vi "MICROMATIC.vi"() -> ()   [LabVIEW 2019]
uses:
  <vilib>/Utility/file.llb/Write Delimited Spreadsheet (string).vi
panel:
  in  "DATA LOGGING":bool
  in  "TEMPERATURE":bool
  out "DATE & TIME":timestamp
  out "Temperature (°C )":dynamicdata(graph)
  in  "SELECT A .CSV FILE TO WRITE DATA":path
  out "Vibration ( µA)":dynamicdata(graph)
  in  "VIBRATION":bool
  # "1.Connect vibration sensor to NI-9234 placed in slot no 2 of NI C-DAQ\n2.Connect RTD sensor to NI-9211 placed in slot no 3 of NI C-DAQ"
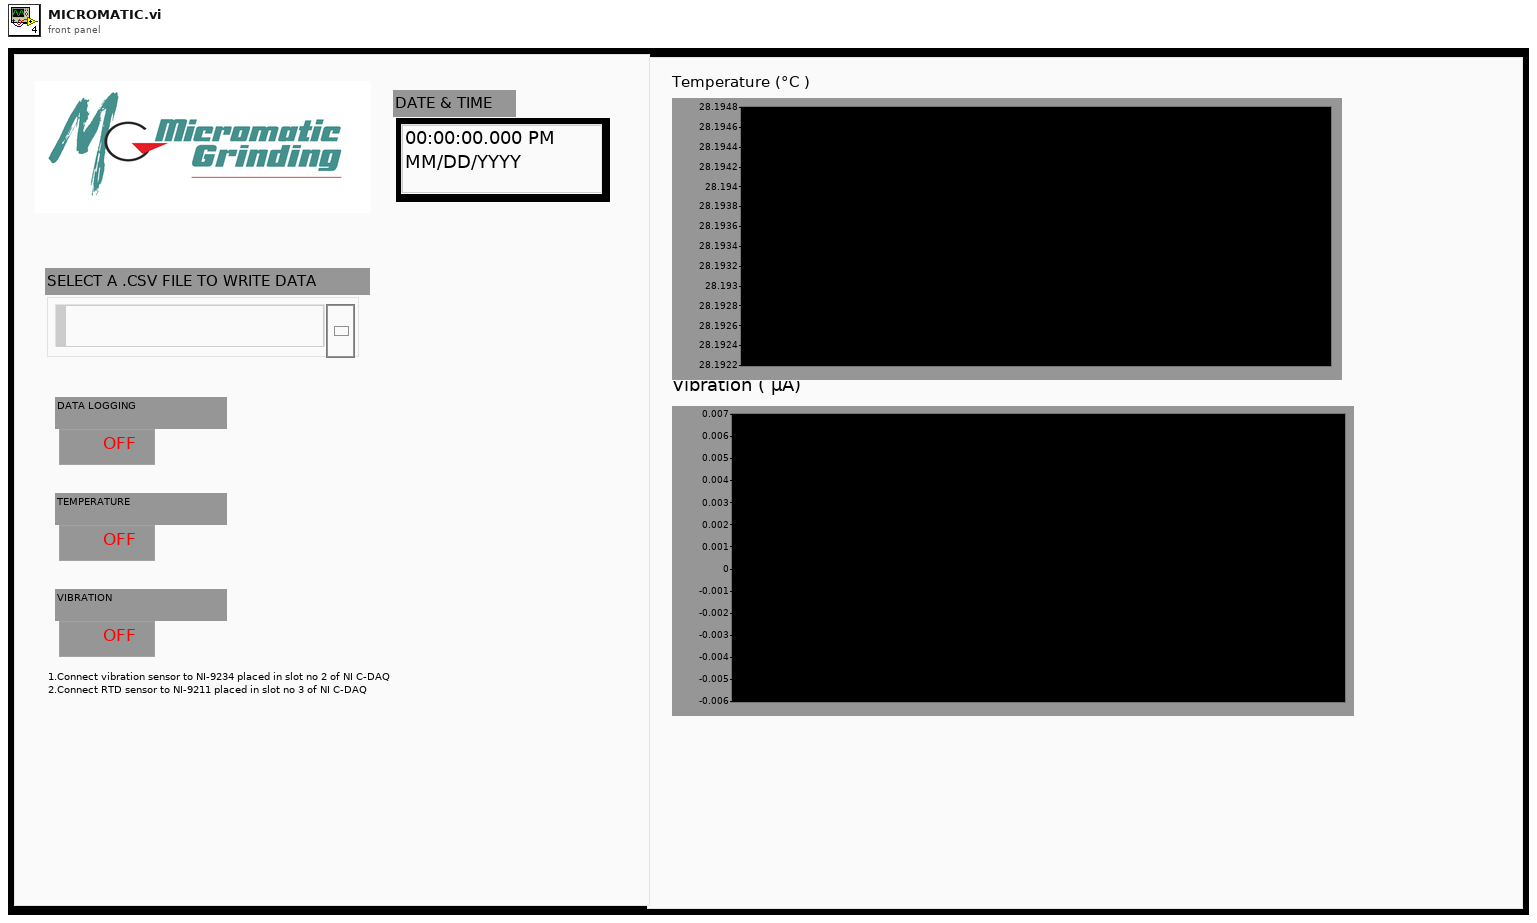
[diagram p1: front panel]
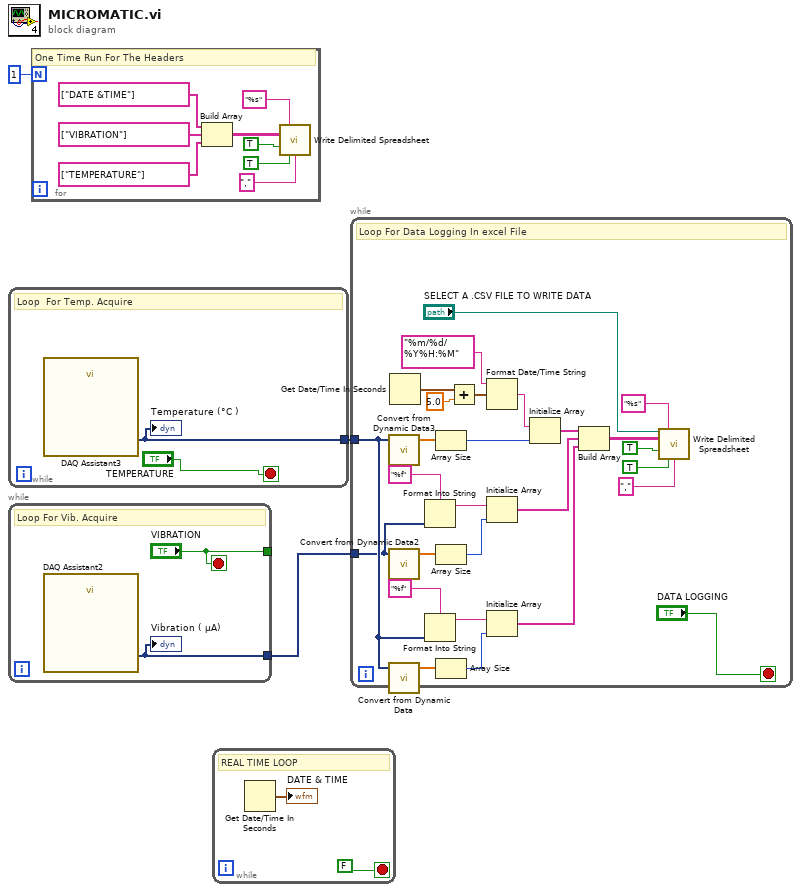
[diagram p0: block diagram]
diagram:
  n1 = while {
    tunnel: [w5] -> w1
    stop <- "TEMPERATURE" stop-if-true
    # "Loop  For Temp. Acquire"
    n2 = call "DAQ Assistant3"() -> ("data"=w5:dynamicdata)  [unwired: 16 in, 3 out]
    "Temperature (°C )" <- w5
  }
  n3 = while {
    tunnel: [w7] -> w2
    tunnel: ["VIBRATION"] -> _
    stop <- "VIBRATION" stop-if-true
    # "Loop For Vib. Acquire"
    n4 = call "DAQ Assistant2"() -> ("data"=w7:dynamicdata)  [unwired: 16 in, 3 out]
    "Vibration ( µA)" <- w7
  }
  n5 = for {
    N: 1 -> [_]
    # "One Time Run For The Headers"
    n6 = Build Array(string[] ["DATE &TIME"], string[] ["VIBRATION"], string[] ["TEMPERATURE"]) -> (w11:string[][])
    n7 = call-poly <vilib>:"Write Delimited Spreadsheet.vi"("format (%s)"="%s", "2D data"=w11, "append to file? (new file:F)"=TRUE, "transpose? (no:F)"=TRUE, "delimiter (\\t)"="," ("delimiter (\\t)")) -> ()  [unwired: 9 in, 2 out]
  }
  n8 = while {
    stop <- FALSE ("TIME") stop-if-true
    # "REAL TIME LOOP"
    n9 = Get Date/Time In Seconds() -> (seconds since 1Jan1904=→"DATE & TIME":timestamp)
  }
  n10 = while {
    tunnel: w1 -> [w20]
    tunnel: w2 -> [w19]
    stop <- "DATA LOGGING" stop-if-true
    # "Loop For Data Logging In excel File"
    n11 = call "Convert from Dynamic Data3"("Dynamic Data Type"=w20) -> ("Array"=w28:dbl[])  [unwired: 3 in]
    n12 = call "Convert from Dynamic Data2"("Dynamic Data Type"=w19) -> ("Array"=w39:dbl[])  [unwired: 3 in]
    n13 = call "Convert from Dynamic Data"("Dynamic Data Type"=w20) -> ("Array"=w41:dbl[])  [unwired: 3 in]
    n14 = Get Date/Time In Seconds() -> (seconds since 1Jan1904=w23:timestamp)
    n15 = Format Into String(format string="%f", w19) -> (resulting string=w38:string)  [unwired: 2 in, 1 out]
    n16 = Format Into String(format string="%f", w20) -> (resulting string=w42:string)  [unwired: 2 in, 1 out]
    n17 = Array Size(array=w28) -> (size(s)=w27:i32)
    n18 = Array Size(array=w39) -> (size(s)=w37:i32)
    n19 = Array Size(array=w41) -> (size(s)=w40:i32)
    n20 = Add(x=w23, y=5.0) -> (x+y=w21:timestamp)
    n21 = Format Date/Time String(time format string (%c)="%m/%d/%Y%H:%M", seconds (now)=w21) -> (date/time string=w29:string)  [unwired: 1 in]
    n22 = Initialize Array(w38, w37) -> (w24:string[])
    n23 = Initialize Array(w42, w40) -> (w25:string[])
    n24 = Initialize Array(w29, w27) -> (w26:string[])
    n25 = Build Array(w26, w24, w25) -> (w35:string[][])
    n26 = call-poly <vilib>:"Write Delimited Spreadsheet.vi"("file path (dialog if empty)"="SELECT A .CSV FILE TO WRITE DATA", "format (%s)"="%s", "2D data"=w35, "append to file? (new file:F)"=TRUE, "transpose? (no:F)"=TRUE, "delimiter (\\t)"="," ("delimiter (\\t)")) -> ()  [unwired: 8 in, 2 out]
  }
